vi "NI6071E.TCP Transaction.vi"(0 "connection ID in":refnum<k5>, 2 "NI6071E Command Cluster":T1, 3 "timeout ms (25000)":i32=25000, 5 "error in":errorcluster) -> (14 "connection ID out":refnum<k5>, 16 "NI6071E Response":T1, 19 "error out":errorcluster)   [LabVIEW 2014, in "NI6071E.lvlib"]
uses:
  NI6071E.lvlib
  NI6071ECommandCluster.ctl
panel:
  out "dt / ms":u32
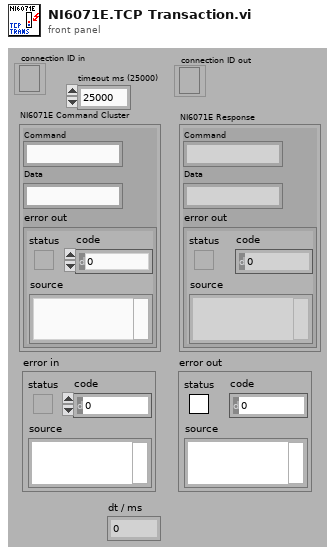
[diagram p1: front panel]
types:
  T1 = typedef "NI6071E.lvlib/NI6071ECommandCluster.ctl" = cluster{"Command":string, "Data":string, "error out":errorcluster}
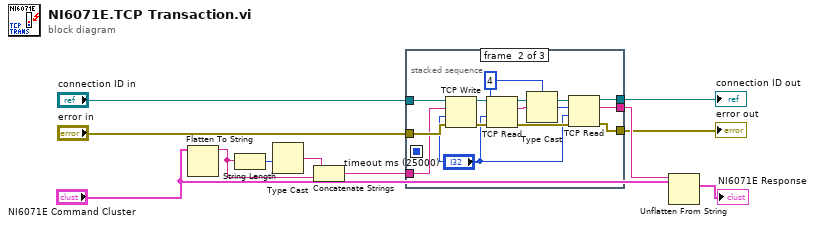
[diagram p0: block diagram]
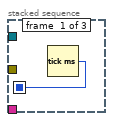
[diagram p2: hidden frame]
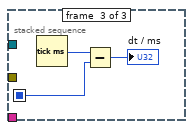
[diagram p3: hidden frame]
diagram:
  n1 = Flatten To String(anything="NI6071E Command Cluster") -> (data string=w8:string)  [unwired: 3 in, 2 out]
  n2 = String Length(string=w8) -> (length=w3:i32)
  n3 = Type Cast(x=w3) -> (*(type *) &x=w4:string)  [unwired: 1 in]
  n4 = Concatenate Strings(w4, w8) -> (w5:string)
  n5 = stacked-sequence {
    seq-local: [w12 _ _] -> [_ _ w28]
    tunnel: "error in" -> [_ w26 _]
    tunnel: [_ w25 _] -> w9
    tunnel: [_ w24 _] -> w7
    tunnel: [_ w23 _] -> w6
    tunnel: w5 -> [_ w15 _]
    tunnel: "connection ID in" -> [_ w14 _]
    frame #0 {
      n6 = Tick Count (ms)() -> (millisecond timer value=w12:u32)
    }
    frame #1 {
      w18 = 4 ("bytes to read")
      n7 = TCP Write(connection ID=w14, data in=w15, error in (no error)=w26, 9:"timeout ms (25000)") -> (connection ID out=w21:refnum<k5>, error out=w22:errorcluster)  [unwired: 1 out]
      n8 = TCP Read(connection ID=w21, bytes to read=w18, error in (no error)=w22, 9:"timeout ms (25000)") -> (connection ID out=w19:refnum<k5>, data out=w16:string, error out=w20:errorcluster)  [unwired: 1 in]
      n9 = Type Cast(type=w18, x=w16) -> (*(type *) &x=w17:i32)
      n10 = TCP Read(connection ID=w19, bytes to read=w17, error in (no error)=w20, 9:"timeout ms (25000)") -> (connection ID out=w23:refnum<k5>, data out=w25:string, error out=w24:errorcluster)  [unwired: 1 in]
    }
    frame #2 {
      n11 = Tick Count (ms)() -> (millisecond timer value=w29:u32)
      n12 = Subtract(x=w29, y=w28) -> (x-y=→"dt / ms":u32)
    }
  }
  "error out" <- w7
  "connection ID out" <- w6
  n13 = Unflatten From String(type="NI6071E Command Cluster", binary string=w9) -> (value=→"NI6071E Response":T1)  [unwired: 3 in, 2 out]
